vi "test Correct Scheduled Labels In Log.vi"(8 "error in":errorcluster, 11 "TestCase in":refnum<class "Logging Loopback.lvclass">) -> (0 "error out":errorcluster, 3 "TestCase out":refnum<class "Logging Loopback.lvclass">)   [LabVIEW 2020, in "Logging Loopback.lvclass"]
uses:
  Logging Loopback.lvclass
  Logging Loopback.lvclass/Logging Loopback.ctl
  6070ecc1-7a7f-4aba-84f3-8f274e3c644e.vi
  <vilib>/WebDAVClient/Advanced/Get Buffer.vi
  <vilib>/addons/_JKI Toolkits/VI Tester/TestCase.llb/TestCase.lvclass
  <vilib>/WebDAVClient/NI_WebDAV.lvlib
  C:/Program Files (x86)/National Instruments/LabVIEW 2020/vi.lib/addons/_JKI Toolkits/VI Tester/TestCase.llb/TestCase.lvclass
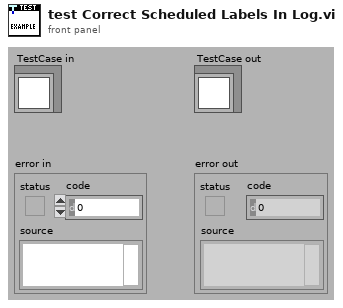
[diagram p1: front panel]
types:
  T1 = typedef "NI_WebDAV.lvlib/SessionHandle.ctl" = refnum<k1>
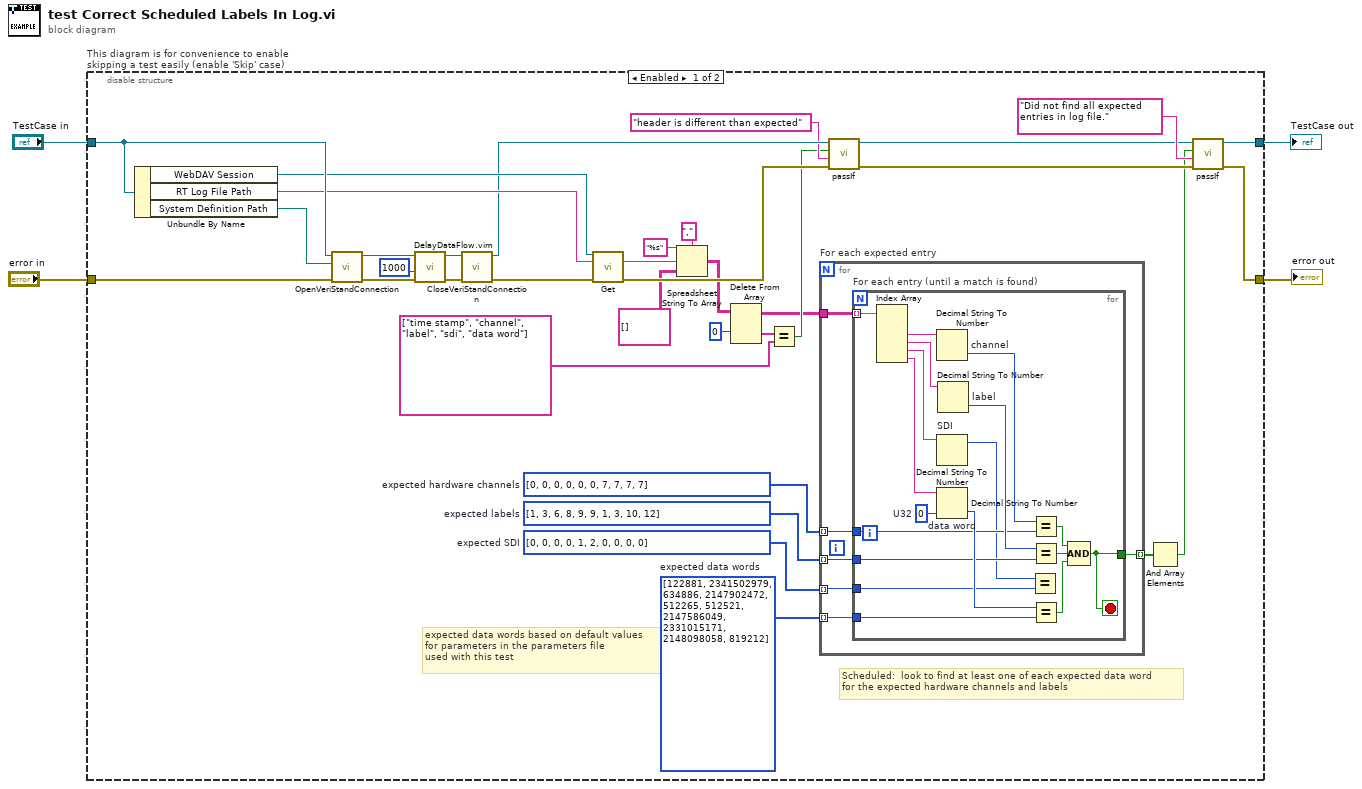
[diagram p0: block diagram]
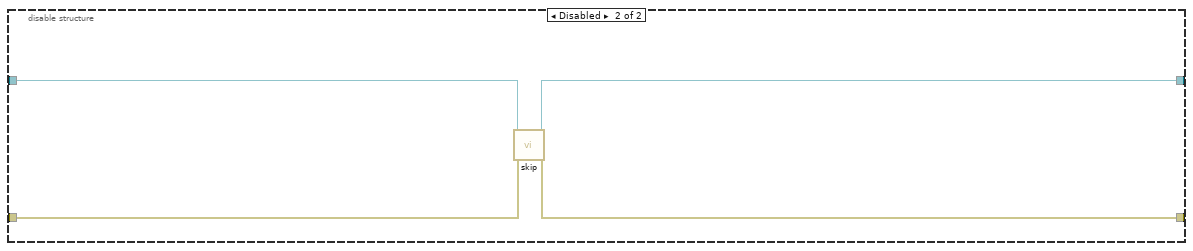
[diagram p2: hidden frame]
diagram:
  n1 = disable-structure "This diagram is for convenience to enable skipping a test easily (enable 'Skip' case)" shown="Enabled" {
    disable-tunnel: "TestCase in" -> [w35 w66]
    disable-tunnel: [w22 w64] -> w1
    disable-tunnel: [w23 w65] -> w3
    disable-tunnel: "error in" -> [w38 w63]
    frame Enabled {
      w5 = i32[] [0, 0, 0, 0, 1, 2, 0, 0, 0, 0]  # expected SDI
      w9 = u32[] [122881, 2341502979, 634886, 2147902472, 512265, 512521, 2147586049, 2331015171, 2148098058, 819212]  # expected data words
      w11 = i32[] [0, 0, 0, 0, 0, 0, 7, 7, 7, 7]  # expected hardware channels
      w10 = i32[] [1, 3, 6, 8, 9, 9, 1, 3, 10, 12]  # expected labels
      # "Scheduled:  look to find at least one of each expected data word\nfor the expected hardware channels and labels"
      # "expected data words based on default values\nfor parameters in the parameters file\nused with this test"
      n2 = Unbundle By Name(w35) -> ("WebDAV Session"=w29:T1, "RT Log File Path"=w28:string, "System Definition Path"=w36:path)
      n3 = call-dynamic "OpenVeriStandConnection.vi"("error in (no error)"=w38, "System Definition File"=w36, "VeriStand Test Case in"=w35) -> ("error out"=w37:errorcluster, "VeriStand Test Case out"=w32:refnum<class "Logging Loopback.lvclass">)  [unwired: 6 in, 1 out]
      n4 = call "DelayDataFlow.vim"("value in"=w37, "milliseconds to wait"=u32 1000) -> ("value out"=w34:errorcluster)  [unwired: 2 in, 1 out]
      n5 = call-dynamic "CloseVeriStandConnection.vi"("error in (no error)"=w34, "VeriStand Test Case in"=w32) -> ("error out"=w31:errorcluster, "VeriStand Test Case out"=w19:refnum<class "Logging Loopback.lvclass">)  [unwired: 8 in]
      n6 = call-poly <vilib>:"Get.vi"("session handle"=w29, "relative uri"=w28, "error in (no error)"=w31) -> ("data"=w27:string, "error out"=w30:errorcluster)  [unwired: 10 in, 1 out]
      n7 = Spreadsheet String To Array(delimiter (Tab)=",", format string="%s", spreadsheet string=w27, array type (2D Dbl)=string[][] []) -> (array=w16:string[][])
      n8 = Delete From Array(array=w16, index (row)=0) -> (deleted portion=w15:string[], array with subset deleted=w8:string[][])  [unwired: 2 in]
      n9 = Equal?(x=w15, y=string[] ["time stamp", "channel", "label", "sdi", "data word"]) -> (x = y?=w12:bool)
      n10 = for "For each expected entry" {
        tunnel: w11 -> [w43] mode=indexing
        tunnel: w10 -> [w42] mode=indexing
        tunnel: w9 -> [w41] mode=indexing
        tunnel: w8 -> [w44]
        tunnel: [w40] -> w7 mode=indexing
        tunnel: w5 -> [w39] mode=indexing
        n11 = for "For each entry (until a match is found)" {
          tunnel: w44 -> [w62] mode=indexing
          tunnel: w43 -> [w55]
          tunnel: w42 -> [w57]
          tunnel: w41 -> [w59]
          tunnel: [w52] -> w40
          tunnel: w39 -> [w45]
          stop <- w52 stop-if-true
          w51 = u32 0  # U32
          n12 = Index Array(array=w62) -> (element #2=w61:string, element #3=w60:string, element #4=w48:string, element #5=w49:string)  [unwired: 5 in, 1 out]
          n13 = Decimal String To Number "channel"(string=w61) -> (number=w54:i32)  [unwired: 2 in, 1 out]
          n14 = Decimal String To Number "SDI"(string=w48) -> (offset past number=w46:i32)  [unwired: 2 in, 1 out]
          n15 = Decimal String To Number "data word"(string=w49, default (0L)=w51) -> (number=w58:u32)  [unwired: 1 in, 1 out]
          n16 = Decimal String To Number "label"(string=w60) -> (number=w56:i32)  [unwired: 2 in, 1 out]
          n17 = Equal?(x=w46, y=w45) -> ()  [unwired: 1 out]
          n18 = Equal?(x=w54, y=w55) -> (x = y?=w50:bool)
          n19 = Equal?(x=w56, y=w57) -> (x = y?=w47:bool)
          n20 = Equal?(x=w58, y=w59) -> (x = y?=w53:bool)
          n21 = Compound Arithmetic op=AND(w50, w47, w53) -> (w52:bool)
        }
      }
      n22 = call-dynamic "passIf.vi"("error in (no error)"=w30, "message (\"\")"="header is different than expected" ("message (\"\")"), "pass"=w12, "TestCase in"=w19) -> ("error out"=w20:errorcluster, "TestCase out"=w18:refnum<class "Logging Loopback.lvclass">)  [unwired: 6 in]
      n23 = And Array Elements(Boolean array=w7) -> (logical AND=w6:bool)
      n24 = call-dynamic "passIf.vi"("error in (no error)"=w20, "message (\"\")"="Did not find all expected entries in log file." ("message (\"\")"), "pass"=w6, "TestCase in"=w18) -> ("error out"=w23:errorcluster, "TestCase out"=w22:refnum<class "Logging Loopback.lvclass">)  [unwired: 6 in]
    }
    frame Disabled {
      # "skip test result while test is under development"
      n25 = call <vilib>:"skip.vi"("error in (no error)"=w63, "TestCase in"=w66) -> ("error out"=w65:errorcluster, "TestCase out"=w64:refnum<class "Logging Loopback.lvclass">)  [unwired: 8 in]
    }
  }
  "error out" <- w3
  "TestCase out" <- w1
